vi "PollEvent.vi"(8 "No Error":errorcluster) -> (0 "error out":errorcluster, 2 "Event Occured?":bool, 3 "Event Binary Data":string)   [LabVIEW 2024, in "SDL3.lvlib" / "Events.lvlib"]
doc: "<B>LV Implementation Note</B>\nSince unions are not availbale in LabVIEW, we send a 128 Bytes cluster in order to recieve event data. The event data is in (probably) little-endian.\n\n<B>Summary</B>\nPoll for currently pending events.\n\n<B>Return Value</B>\n(bool) Returns true if this got an event or false if there are none available.\n\n<B>Remarks</B>\nIf event is not NULL, the next event is removed from the queue and stored in the SDL_Event structure pointed to by event. The 1 returned refers to this event, immediately stored in the SDL Event structure -- not an event to follow.\n\nIf event is NULL, it simply returns 1 if there is an event in the queue, but will not remove it from the queue.\n\nAs this function may implicitly call SDL_PumpEvents(), you can only call this function in the thread that set the video mode.\n\nSDL_PollEvent() is the favored way of receiving system events since it can be done from the main loop and does not suspend the main loop while waiting on an event to be posted."
uses:
  Events.lvlib
  Lib/SDL3-32.dll
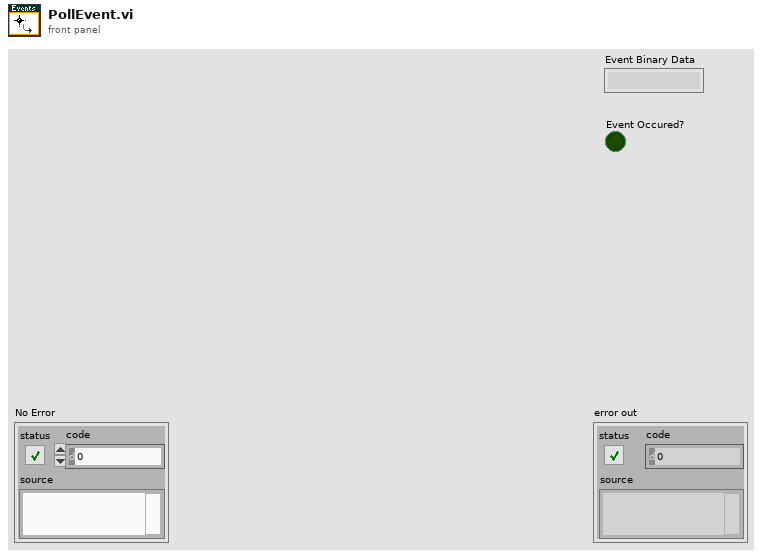
[diagram p1: front panel]
types:
  T1 = cluster{u8, u8, u8, u8, u8, u8, u8, u8, u8, u8, u8, u8, u8, u8, u8, u8, u8, u8, u8, u8, u8, u8, u8, u8, u8, u8, u8, u8, u8, u8, u8, u8, u8, u8, u8, u8, u8, u8, u8, u8, u8, u8, u8, u8, u8, u8, u8, u8, u8, u8, u8, u8, u8, u8, u8, u8, u8, u8, u8, u8, u8, u8, u8, u8, u8, u8, u8, u8, u8, u8, u8, u8, u8, u8, u8, u8, u8, u8, u8, u8, u8, u8, u8, u8, u8, u8, u8, u8, u8, u8, u8, u8, u8, u8, u8, u8, u8, u8, u8, u8, u8, u8, u8, u8, u8, u8, u8, u8, u8, u8, u8, u8, u8, u8, u8, u8, u8, u8, u8, u8, u8, u8, u8, u8, u8, u8, u8, u8}
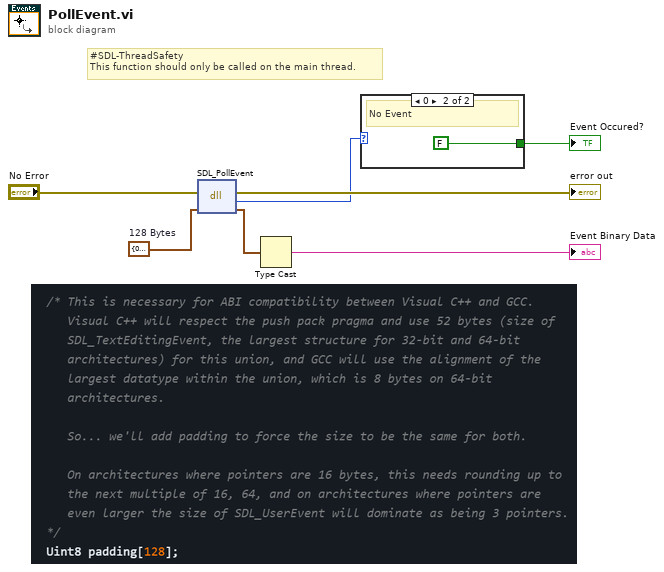
[diagram p0: block diagram]
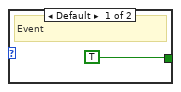
[diagram p2: hidden frame]
diagram:
  w1 = T1 {0, 0, 0, 0, 0, 0, 0, 0, 0, 0, 0, 0, 0, 0, 0, 0, 0, 0, 0, 0, 0, 0, 0, 0, 0, 0, 0, 0, 0, 0, 0, 0, 0, 0, 0, 0, 0, 0, 0, 0, 0, 0, 0, 0, 0, 0, 0, 0, 0, 0, 0, 0, 0, 0, 0, 0, 0, 0, 0, 0, 0, 0, 0, 0, 0, 0, 0, 0, 0, 0, 0, 0, 0, 0, 0, 0, 0, 0, 0, 0, 0, 0, 0, 0, 0, 0, 0, 0, 0, 0, 0, 0, 0, 0, 0, 0, 0, 0, 0, 0, 0, 0, 0, 0, 0, 0, 0, 0, 0, 0, 0, 0, 0, 0, 0, 0, 0, 0, 0, 0, 0, 0, 0, 0, 0, 0, 0, 0}  # 128 Bytes
  # "#SDL-ThreadSafety\nThis function should only be called on the main thread."
  n1 = dll-call lib="C:/Users/Thomas/Documents/Projects/LV-SDL3/Lib/SDL3-*.*" fn="SDL_PollEvent"(error in="No Error", "event"=w1) -> (error out=→"error out":errorcluster, "return type"=w3:i32, "event"=w2:T1)  [unwired: 2 in, 1 out]
  n2 = Type Cast(x=w2) -> (*(type *) &x=→"Event Binary Data":string)  [unwired: 1 in]
  n3 = case shown="0" w3 {
    tunnel: [TRUE FALSE] -> w5
    frame Default {
      # "Event"
    }
    frame 0 {
      # "No Event"
    }
  }
  "Event Occured?" <- w5
